vi "Log Results.vi"(8 "error in (no error)":errorcluster, 10 "Result":refnum<class "Mag Lab Result.lvclass">, 11 "Common Measurements in":refnum<class "Common Measurements.lvclass">) -> (0 "error out":errorcluster, 3 "Common Measurements out":refnum<class "Common Measurements.lvclass">)   [LabVIEW 2015, in "Common Measurements.lvclass"]
uses:
  Common Measurements.lvclass
  Mag Lab Result/Mag Lab Result.lvclass
  Common Measurements.lvclass/Common Measurements.ctl
  Mag Lab Root/Mag Lab Root.lvclass/Mag Lab Root.ctl
  Mag Lab Result/Mag Lab Result.lvclass/Mag Lab Result.ctl
  Mag Lab Measure Base/Mag Lab Measure Base.lvclass/Mag Lab Measure Base.ctl
  MagLabGraph Messages/File updated Msg/File updated Msg.lvclass/File updated Msg.ctl
  <vilib>/ActorFramework/Message Enqueuer/Message Enqueuer.lvclass/Message Enqueuer.ctl
  <vilib>/ActorFramework/Message Enqueuer/Enqueue.vi
  <vilib>/ActorFramework/Message Priority Queue/Priority Enqueue.vi
  <vilib>/ActorFramework/Message Enqueuer/Message Enqueuer.lvclass
  MagLabGraph Messages/File updated Msg/File updated Msg.lvclass
  Mag Lab Measure Base/Mag Lab Measure Base.lvclass
  Mag Lab Root/Mag Lab Root.lvclass
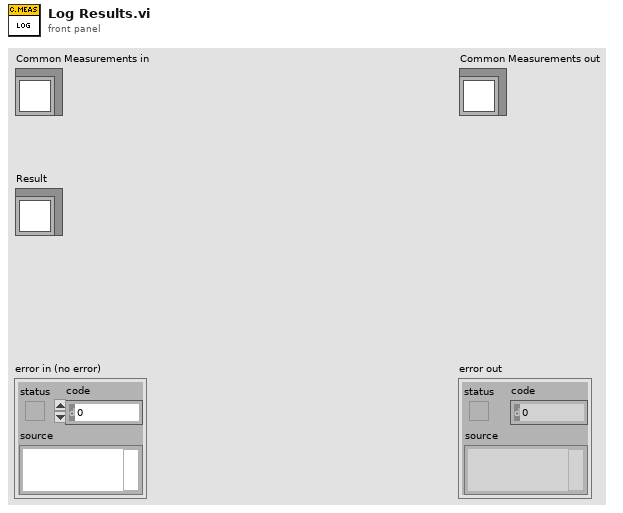
[diagram p1: front panel]
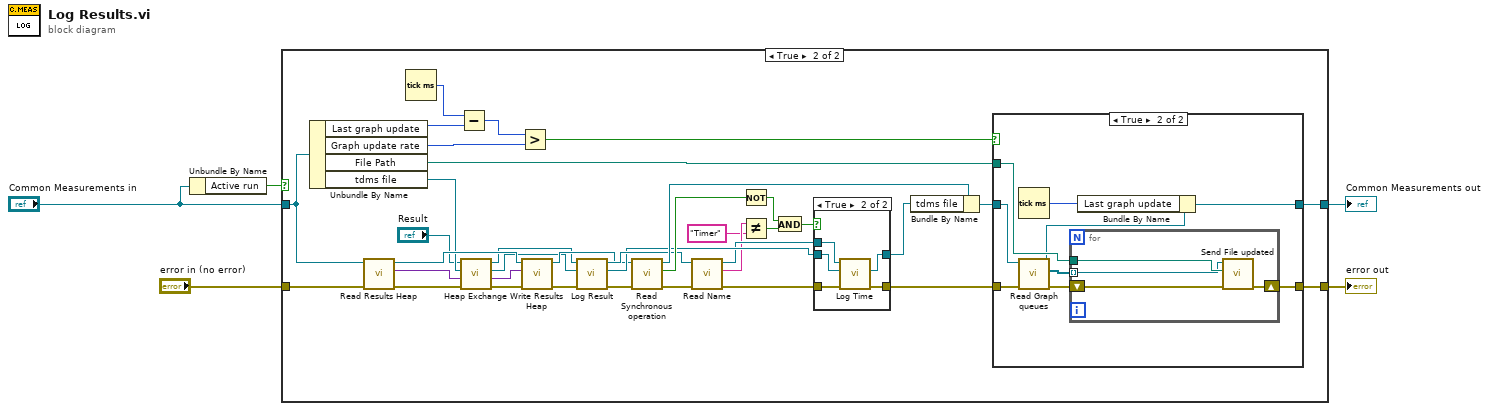
[diagram p0: block diagram]
diagram:
  n1 = Unbundle By Name("Common Measurements in") -> ("Active run"=w5:bool)
  n2 = case shown="True" w5 {
    tunnel: "error in (no error)" -> [w7 w19]
    tunnel: [w7 w35] -> w3
    tunnel: "Common Measurements in" -> [w6 w44]
    tunnel: [w6 w41] -> w1
    frame False {
    }
    frame True {
      n3 = Unbundle By Name(w44) -> ("Last graph update"=w39:u32, "Graph update rate"=w37:u32, "File Path"=w42:path, "tdms file"=w14:refnum<k34>)
      n4 = call "Read Results Heap.vi"("error in (no error)"=w19, "Mag Lab Root in"=w44) -> ("error out"=w17:errorcluster, "Results Heap"=w16:variant, "Mag Lab Root out"=w20:refnum<class "Common Measurements.lvclass">)  [unwired: 7 in]
      n5 = Tick Count (ms)() -> (millisecond timer value=w40:u32)
      n6 = Subtract(x=w40, y=w39) -> (x-y=w38:u32)
      n7 = call-dynamic "Heap Exchange.vi"("error in (no error)"=w17, "Results Heap"=w16, "tdms file"=w14, "Mag Lab Result in"="Result") -> ("error out"=w10:errorcluster, "Results Heap out"=w15:variant, "tdms file out"=w13:refnum<k34>, "Mag Lab Result out"=w11:refnum<class "Mag Lab Result.lvclass">)  [unwired: 4 in]
      n8 = Greater?(x=w38, y=w37) -> (0:w36:bool)
      n9 = call "Write Results Heap.vi"("error in (no error)"=w10, "Results Heap"=w15, "Mag Lab Root in"=w20) -> ("error out"=w9:errorcluster, "Mag Lab Root out"=w18:refnum<class "Common Measurements.lvclass">)  [unwired: 7 in]
      n10 = call-dynamic "Log Result.vi"("error in (no error)"=w9, "tdms file"=w13, "Mag Lab Result in"=w11) -> ("error out"=w8:errorcluster, "tdms file out"=w30:refnum<k34>, "Mag Lab Result out"=w31:refnum<class "Mag Lab Result.lvclass">)  [unwired: 6 in]
      n11 = call "Read Synchronous operation.vi"("error in (no error)"=w8, "Mag Lab Root in"=w18) -> ("error out"=w27:errorcluster, "Synchronous operation"=w33:bool, "Mag Lab Root out"=w34:refnum<class "Common Measurements.lvclass">)  [unwired: 7 in]
      n12 = call "Read Name.vi"("error in (no error)"=w27, "Mag Lab Result in"=w31) -> ("error out"=w26:errorcluster, "Name"=w25:string, "Mag Lab Result out"=w28:refnum<class "Mag Lab Result.lvclass">)  [unwired: 7 in]
      n13 = Not(x=w33) -> (.not. x?=w23:bool)
      n14 = Not Equal?(x=w25, y="Timer") -> (x != y?=w22:bool)
      n15 = And(x=w23, y=w22) -> (x .and. y?=w21:bool)
      n16 = case shown="True" w21 {
        tunnel: w26 -> [w46 w51]
        tunnel: [w46 w50] -> w32
        tunnel: w28 -> [_ w49]
        tunnel: w30 -> [w45 w48]
        tunnel: [w45 w47] -> w29
        frame False {
        }
        frame True {
          n17 = call-dynamic "Log Time.vi"("error in (no error)"=w51, "tdms file"=w48, "Mag Lab Result in"=w49) -> ("error out"=w50:errorcluster, "tdms file out"=w47:refnum<k34>)  [unwired: 6 in, 1 out]
        }
      }
      n18 = Bundle By Name(cluster=w34, "tdms file"=w29) -> (w43:refnum<class "Common Measurements.lvclass">)
      n19 = case shown="True" w36 {
        tunnel: w43 -> [w53 w62]
        tunnel: w42 -> [_ w61]
        tunnel: [w53 w58] -> w41
        tunnel: w32 -> [w52 w56]
        tunnel: [w52 w54] -> w35
        frame False {
        }
        frame True {
          n20 = Tick Count (ms)() -> (millisecond timer value=w57:u32)
          n21 = call "Read Graph queues.vi"("error in (no error)"=w56, "Mag Lab Measure Base in"=w62) -> ("error out"=w55:errorcluster, "Graph queues"=w59:refnum<class "Message Enqueuer.lvclass">[], "Mag Lab Measure Base out"=w60:refnum<class "Common Measurements.lvclass">)  [unwired: 7 in]
          n22 = for {
            tunnel: w61 -> [w66]
            tunnel: w59 -> [w65] mode=indexing
            shift-right: [w63] -> w54
            shift-left: w55 -> [w64]
            n23 = call "Send File updated.vi"("error in (no error)"=w64, "File Path Control"=w66, "Message Enqueuer"=w65) -> ("error out"=w63:errorcluster)  [unwired: 7 in, 1 out]
          }
          n24 = Bundle By Name(cluster=w60, "Last graph update"=w57) -> (w58:refnum<class "Common Measurements.lvclass">)
        }
      }
    }
  }
  "error out" <- w3
  "Common Measurements out" <- w1
